vi "All_Demos.vi"() -> ()   [LabVIEW 2011]
uses:
  VIremote.llb/VIremoteFunction.ctl
  VIremote.llb/VIremoteNavigationBar.ctl
  VIremote.llb/VIremoteStatus.ctl
panel:
  in  "Use emulation":bool=TRUE
  in  "Make Palette":bool
  in  "Select demo ring":i16(ring)=14 caption="Select Demo" items=["Demo String and Numeric.vi", "Demo Navigation Bar.vi", "Demo UI Orientation.vi", "Demo Dialog.vi", "Demo Ring and Enum.vi", "Demo Combo Box.vi", "Demo Slider.vi", "Demo Date and Time.vi", "Demo User Notification and Status.vi", "Demo Accelerometer Graph.vi", "Demo Multitouch.vi", "Demo Simple Sound.vi", "Demo File Dialog.vi", "Demo Scrolling.vi", "-", "QUIT"]
  in  "stop":bool
  out "IP address of\nthis computer":string
  # "If this is the first time you run this then follow the instructions below. The free version only stay connected for 2 minutes but  there is an exe file with these demos in the folder VIremoteFree30min.  The exe will let the demo run for 30 minutes.\n\nRun This VI.\nStart VIremote on your iOS device.\nEnter the IP address of this computer (see below) on the info page. Tap \"Connect\".\nThis VI will show on the screen and a table will be presented where you can select a demo to try out.\n\nView the diagram of this and all the demos to learn more. Documentation can be found in the doc folder (use the HelpBrowser.vi).\n\nUse the Add Palettes button below to add VIremote palettes to the Controls and Functions Palette sets. Use Add Palettes again when a new version is released.\n\nSend feedback and questions to iPhone@throwlab.com \n\nDon't forget to write a review on the App Store  if you like it.\n/ThrowLab"
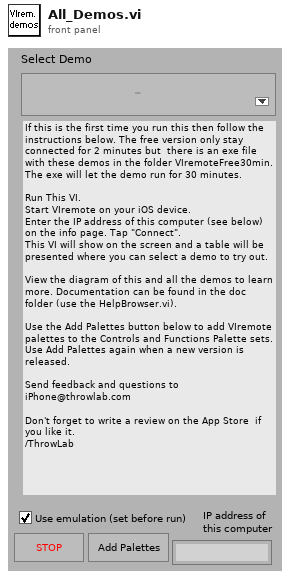
[diagram p1: front panel]
types:
  T1 = typedef "VIremoteNavigationBar.ctl" = enum16{"Show Bar", "Hide Bar", "Clear History", "Set Bar Tint Color", "Set Bar Title", "Set Bar Prompt", "Show Back Button", "Hide Back Button", "Set Back Button Text", "Add Right Button", "Add Left Button", "Remove Button"}
  T2 = typedef "VIremoteFunction.ctl" = enum16{"Do nothing", "Stop controller", "Close this connection", "Show info panel", "Set VI to control", "Set Accelerometer freq (Hz)", "Show Alert message", "Start Sound Input", "Stop Sound Input", "Set Volume (0-100)", "Set sound output Speaker", "Set sound output Receiver", "Play Sound", "Repeat Sound", "Stop Sound", "Pause Sound", "Resume Sound", "Set panel width of caller (320 or 480)", "Set Panel Size to Portrait", "Set Panel Size to Landscape", "Set Panel Size as Current Orientation", "Allow all UI Orientations", "Send user notification", "Disable Scrolling", "Normal Scrolling", "Page Scrolling", "Set Scroll Offset", "Page Indicator Position"}
  T3 = typedef "VIremoteStatus.ctl" = enum16{"Connected BOOL", "Number of connections DBL", "VIremoteController ver.", "VIremote ver. DBL", "Screen width DBL", "Screen height DBL", "Current navigation bar height DBL", "Current UI orientation", "Background supported BOOL", "Background state BOOL", "Device UI idiom (0=phone,1=iPad) DBL", "Device name", "Device unique id", "Device system ver.", "Device model", "Device HW model"}
  T4 = typedef "VIremoteInit.ctl" = cluster{"port (2055)":u16, "Use mouse emulation (T)":bool, "Use keyboard emulation (T)":bool, "Allow multiple connections (F)":bool, "Debug mode/error dialog (F)":bool, "Temporary directory (default)":path, "Mouse emulation VI path":path, "Keyboard emulation VI path":path, "Enable VI Select button(T)":bool, "Enable auto scroll(T)":bool}
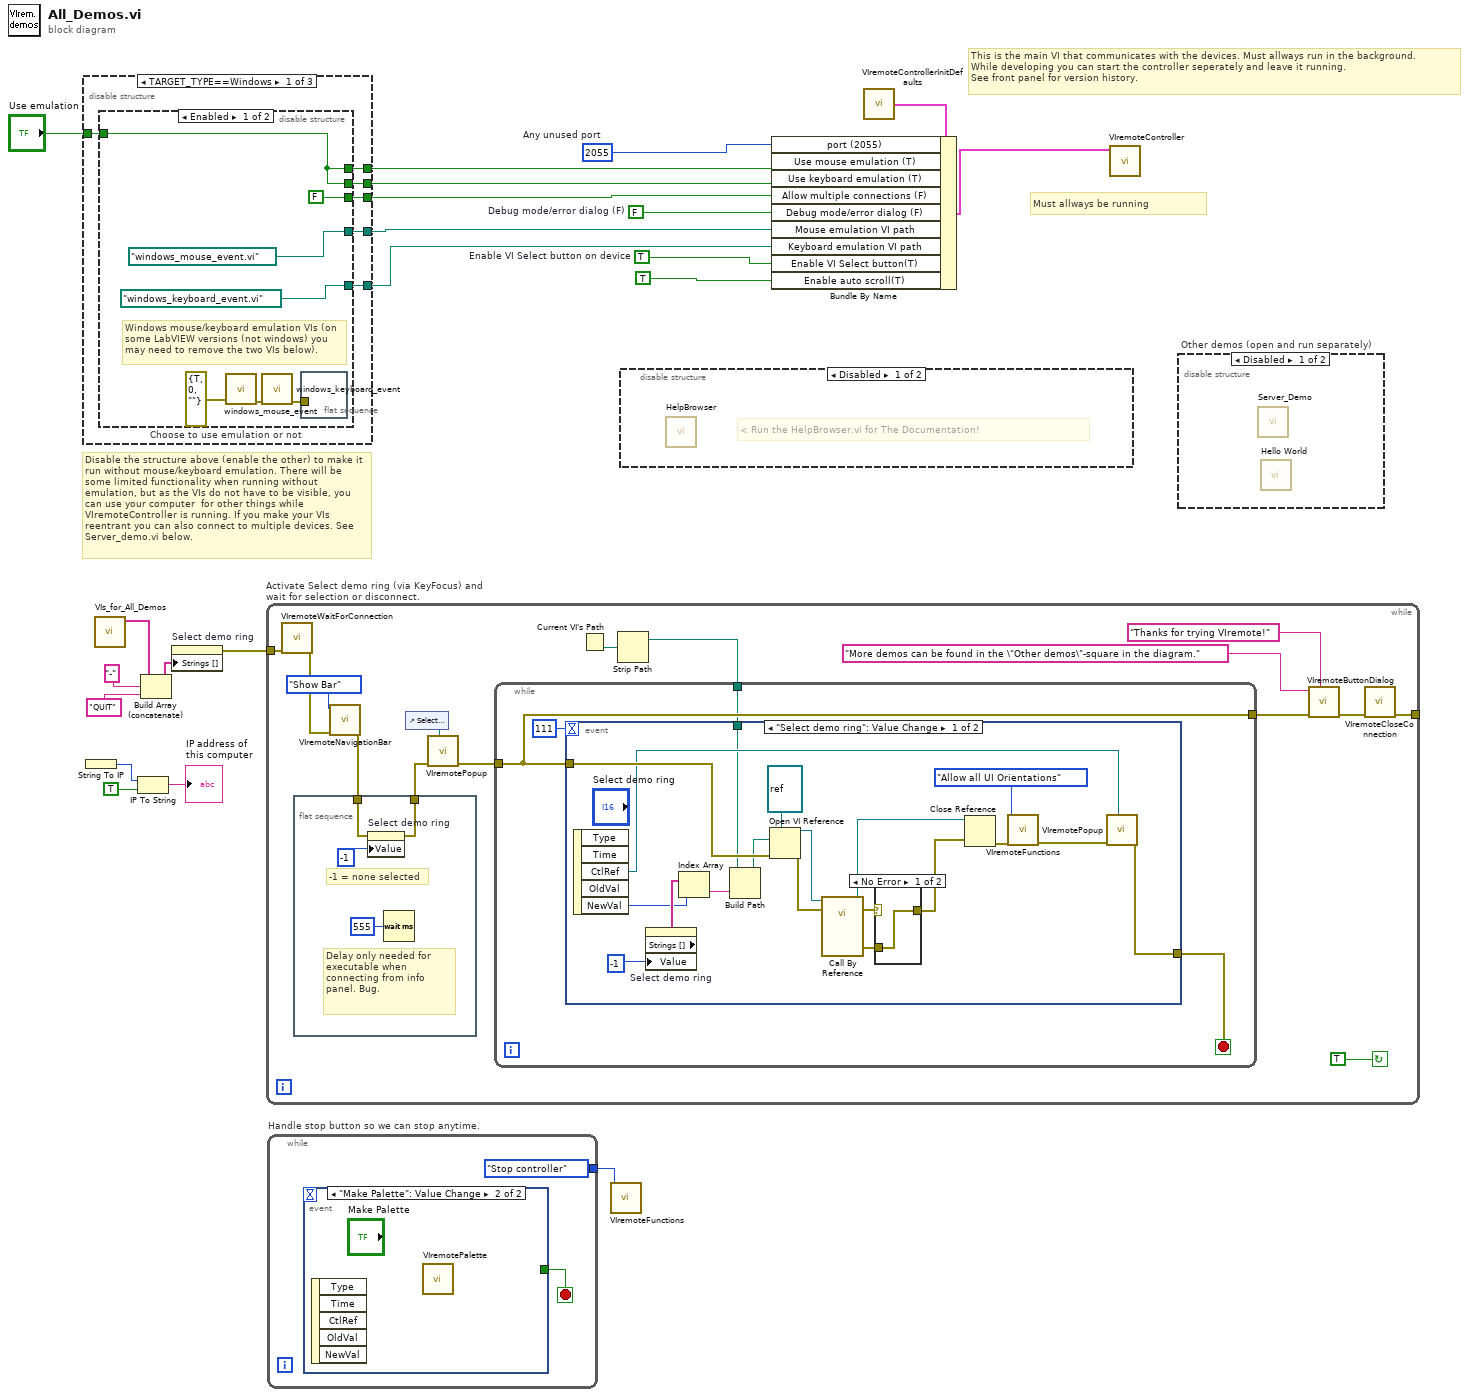
[diagram p0: block diagram]
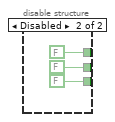
[diagram p3: hidden frame]
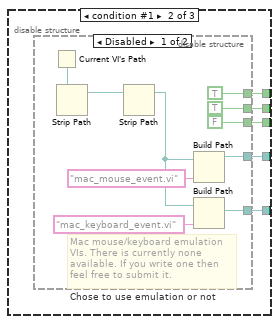
[diagram p4: hidden frame]
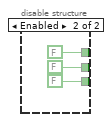
[diagram p5: hidden frame]
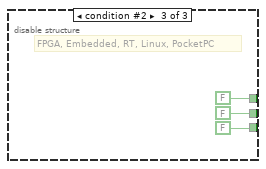
[diagram p6: hidden frame]
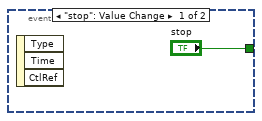
[diagram p7: hidden frame]
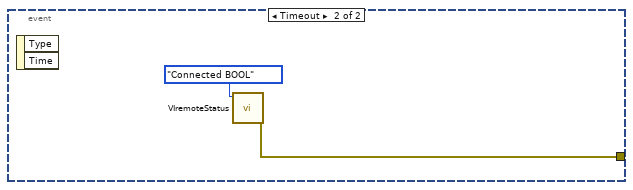
[diagram p9: hidden frame]
diagram:
  w9 = TRUE  # Enable VI Select button on device
  w17 = FALSE  # Debug mode/error dialog (F)
  w18 = u16 2055  # Any unused port
  # "< Run the HelpBrowser.vi for The Documentation!"
  # "Disable the structure above (enable the other) to make it run without mouse/keyboard emulation. There will be some limited functionality when running without emulation, but as the VIs do not have to be visible, you can use your computer  for other things while VIremoteController is running. If you make your VIs reentrant you can also connect to multiple devices. See Server_demo.vi below."
  # "Must allways be running"
  # "This is the main VI that communicates with the devices. Must allways run in the background.\nWhile developing you can start the controller seperately and leave it running.\nSee front panel for version history."
  n1 = disable-structure shown="TARGET_TYPE==Windows" {
    disable-tunnel: [w27 w42 _] -> w15
    disable-tunnel: [w26 w41 _] -> w14
    disable-tunnel: [w25 w40 FALSE ("Use mouse emulation (T)")] -> w12
    disable-tunnel: [w24 w39 FALSE ("Use keyboard emulation (T)")] -> w11
    disable-tunnel: [w23 w38 FALSE ("Allow multiple connections (F)")] -> w10
    disable-tunnel: "Use emulation" -> [w22 _ _]
    frame condition #0 (active) {
      n2 = disable-structure "Choose to use emulation or not" shown="Enabled" {
        disable-tunnel: [path "windows_mouse_event.vi" ("name or relative path") _] -> w27
        disable-tunnel: [path "windows_keyboard_event.vi" ("name or relative path") _] -> w26
        disable-tunnel: [w30 FALSE ("Use mouse emulation (T)")] -> w25
        disable-tunnel: [w30 FALSE ("Use keyboard emulation (T)")] -> w24
        disable-tunnel: [FALSE ("Allow multiple connections (F)") FALSE ("Allow multiple connections (F)")] -> w23
        disable-tunnel: w22 -> [w30 _]
        frame Enabled {
          # "Windows mouse/keyboard emulation VIs (on some LabVIEW versions (not windows) you may need to remove the two VIs below)."
          n3 = call "windows_mouse_event.vi"("error in (no error)"=errorcluster {"status"=TRUE, "code"=0, "source"=""}) -> ("error out"=w32:errorcluster)  [unwired: 4 in, 6 out]
          n4 = call "windows_keyboard_event.vi"("error in (no error)"=w32) -> ("error out"=w31:errorcluster)  [unwired: 1 in, 9 out]
          n5 = flat-sequence {
            tunnel: w31 -> [_]
            frame #0 {
            }
          }
        }
        frame Disabled {
        }
      }
    }
    frame condition #1 {
      n6 = disable-structure "Chose to use emulation or not" shown="Disabled" {
        disable-tunnel: [w47 _] -> w42
        disable-tunnel: [w46 _] -> w41
        disable-tunnel: [TRUE ("Use mouse emulation (T)") FALSE ("Use mouse emulation (T)")] -> w40
        disable-tunnel: [TRUE ("Use keyboard emulation (T)") FALSE ("Use keyboard emulation (T)")] -> w39
        disable-tunnel: [FALSE ("Allow multiple connections (F)") FALSE ("Allow multiple connections (F)")] -> w38
        frame Disabled {
          # "Mac mouse/keyboard emulation VIs. There is currently none available. If you write one then feel free to submit it."
          n7 = Current VI's Path() -> (path=w44:path)
          n8 = Strip Path(path=w44) -> (stripped path=w45:path)  [unwired: 1 out]
          n9 = Strip Path(path=w45) -> (stripped path=w43:path)  [unwired: 1 out]
          n10 = Build Path(base path=w43, name or relative path="mac_mouse_event.vi") -> (appended path=w47:path)
          n11 = Build Path(base path=w43, name or relative path="mac_keyboard_event.vi") -> (appended path=w46:path)
        }
        frame Enabled {
        }
      }
    }
    frame condition #2 {
      # "FPGA, Embedded, RT, Linux, PocketPC"
    }
  }
  n12 = String To IP() -> (0:w21:u32)  [unwired: 1 out]
  n13 = call "VIs_for_All_Demos.vi"() -> ("Strings []"=w7:string[])  [unwired: 1 in, 10 out]
  n14 = IP To String(1:TRUE ("dot notation? (F)"), 2:w21) -> (0:→"IP address of\nthis computer":string)
  n15 = Build Array (concatenate)(w7, "-", "QUIT") -> (w6:string[])
  n16 = property on="Select demo ring" class="Ring (strict)"("Strings []"=w6) -> (error out=w8:errorcluster)  [unwired: 2 in, 1 out]
  n17 = while "Activate Select demo ring (via KeyFocus) and wait for selection or disconnect." {
    tunnel: [w72] -> _
    tunnel: w8 -> [w68]
    stop <- TRUE continue-if-true
    n18 = call "VIremoteWaitForConnection.vi"("error in (no error)"=w68) -> ("error out"=w61:errorcluster)  [unwired: 10 out]
    n19 = flat-sequence {
      tunnel: [w76] -> w66
      tunnel: w62 -> [w75]
      frame #0 {
        # "Delay only needed for executable when connecting from info panel. Bug."
        # "-1 = none selected"
        n20 = property on="Select demo ring" class="Ring (strict)"(error in=w75, "Value"=-1) -> (error out=w76:errorcluster)  [unwired: 1 in, 1 out]
        n21 = Wait (ms)(milliseconds to wait=u32 555) -> ()  [unwired: 1 out]
      }
    }
    n22 = call "VIremoteNavigationBar.vi"("error in (no error)"=w61, "Func"=VIremoteNavigationBar."Show Bar") -> ("error out"=w62:errorcluster)  [unwired: 3 in, 6 out]
    n23 = control-ref of="Select demo ring"() -> (w64:refnum<vi>)
    n24 = call "VIremotePopup.vi"("Control Refnum"=w64, "error in (no error)"=w66) -> ("error out"=w63:errorcluster)  [unwired: 1 in, 8 out]
    n25 = Current VI's Path() -> (path=w60:path)
    n26 = Strip Path(path=w60) -> (stripped path=w59:path)  [unwired: 1 out]
    n27 = while {
      tunnel: w63 -> [w79]
      tunnel: [w79] -> w67
      tunnel: w59 -> [w78]
      stop <- w80 stop-if-true
      n28 = event shown="[0] \"Select demo ring\": Value Change" {
        selector: _ -> [_ _]
        dyn-events: _ -> [_ _]
        timeout: 111 -> [_ _]
        tunnel: [w86 w103] -> w80
        tunnel: w79 -> [w91 _]
        tunnel: w78 -> [w83 _]
        event "Select demo ring": Value Change {
          n29 = event-data() -> ("CtlRef"=w87:refnum<vi>, "NewVal"=w99:i16)  [unwired: 4 out]
          n30 = property on="Select demo ring" class="Ring (strict)"("Value"=-1) -> ("Strings []"=w100:string[])  [unwired: 2 in, 2 out]
          n31 = Index Array(array=w100, index=w99) -> (element=w82:string)
          n32 = Build Path(base path=w83, name or relative path=w82) -> (appended path=w84:path)
          n33 = Open VI Reference(type specifier VI Refnum (for type only)=refnum<vi> refnum, vi path=w84, error in (no error)=w91) -> (vi reference=w98:refnum<vi>, error out=w95:errorcluster)  [unwired: 3 out]
          n34 = call-by-ref "?"(reference=w98, error in=w95) -> (reference out=w96:refnum<vi>, error out=w94:errorcluster, 0:"error out"=w93:errorcluster)  [unwired: 11 in]
          n35 = case shown="No Error" w94 {
            selector: w94 -> [_ w102]
            tunnel: w93 -> [w101 _]
            tunnel: [w101 w102] -> w92
            frame No Error {
            }
            frame Error {
            }
          }
          n36 = Close Reference(reference=w96, error in (no error)=w92) -> (error out=w89:errorcluster)
          n37 = call "VIremoteFunctions.vi"("error in (no error)"=w89, "Function"=VIremoteFunction."Allow all UI Orientations") -> ("error out"=w85:errorcluster)  [unwired: 4 in, 5 out]
          n38 = call "VIremotePopup.vi"("Control Refnum"=w87, "error in (no error)"=w85) -> ("error out"=w86:errorcluster)  [unwired: 9 out]
        }
        event Timeout {
          n39 = event-data() -> ()  [unwired: 3 out]
          n40 = call "VIremoteStatus.vi"("Status item"=VIremoteStatus."Connected BOOL") -> ("error out"=w103:errorcluster)  [unwired: 2 in, 8 out]
        }
      }
    }
    n41 = call "VIremoteButtonDialog.vi"("Window Title (\"\")"="Thanks for trying VIremote!" ("message"), "error in (no error)"=w67, "message"="More demos can be found in the \"Other demos\"-square in the diagram.") -> ("error out"=w70:errorcluster)  [unwired: 1 in, 7 out]
    n42 = call "VIremoteCloseConnection.vi"("error in (no error)"=w70) -> ("error out"=w72:errorcluster)  [unwired: 1 in, 9 out]
  }
  n43 = while "Handle stop button so we can stop anytime." {
    tunnel: [VIremoteFunction."Stop controller" ("Function")] -> w13
    stop <- w106 stop-if-true
    n44 = event shown="[1] \"Make Palette\": Value Change" {
      selector: _ -> [_ _]
      dyn-events: _ -> [_ _]
      timeout: _ -> [_ _]
      tunnel: ["stop" _] -> w106
      event "stop": Value Change {
        n45 = event-data() -> ()  [unwired: 4 out]
      }
      event "Make Palette": Value Change {
        n46 = event-data() -> ()  [unwired: 6 out]
        n47 = call "VIremotePalette.vi"() -> ()  [unwired: 1 out]
      }
    }
  }
  n48 = call "VIremoteFunctions.vi"("Function"=w13) -> ()  [unwired: 5 in, 6 out]
  n49 = disable-structure shown="Disabled" {
    frame Disabled {
      n50 = call "HelpBrowser.vi"() -> ()  [unwired: 1 in]
    }
    frame Enabled {
    }
  }
  n51 = call "VIremoteControllerInitDefaults.vi"() -> ("Init defaults"=w2:T4)
  n52 = Bundle By Name(cluster=w2, "port (2055)"=w18, "Use mouse emulation (T)"=w12, "Use keyboard emulation (T)"=w11, "Allow multiple connections (F)"=w10, "Debug mode/error dialog (F)"=w17, "Mouse emulation VI path"=w15, "Keyboard emulation VI path"=w14, "Enable VI Select button(T)"=w9, "Enable auto scroll(T)"=TRUE) -> (w16:T4)
  n53 = call "VIremoteController.vi"("Init (can't be changed while running)"=w16) -> ()  [unwired: 11 out]
  n54 = disable-structure "Other demos (open and run separately)" shown="Disabled" {
    frame Disabled {
      n55 = call "Server_Demo.vi"() -> ()  [unwired: 1 out]
      n56 = call "Hello World.vi"() -> ()  [unwired: 1 in]
    }
    frame Enabled {
    }
  }
